vi "GetSoftwareLimits.vi"(8 "error in (no error)":errorcluster, 11 "VISA resource name":refnum<visa-resource-name>="COM15") -> (0 "error out":errorcluster, 2 "Right limit":dbl, 3 "Left limit":dbl)   [LabVIEW 2013]
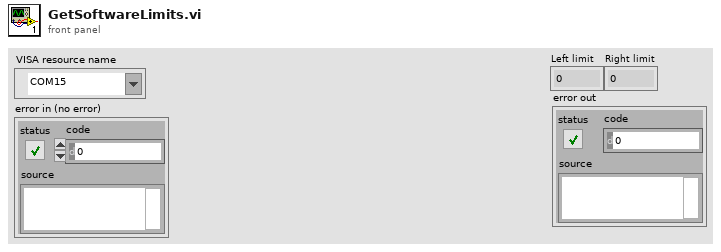
[diagram p1: front panel]
types:
  T1 = cluster{"VISA resource name":refnum<visa-resource-name>, "Device name":string, "Controller address":i32, "error":errorcluster}
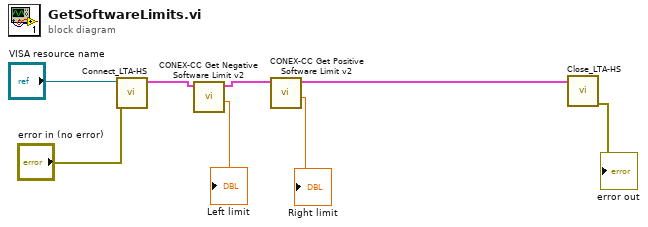
[diagram p0: block diagram]
diagram:
  n1 = call "Connect_LTA-HS.vi"("error in (no error)"="error in (no error)", "VISA resource name"="VISA resource name") -> ("Device Connection Cluster"=w7:T1)  [unwired: 8 in, 1 out]
  n2 = call "CONEX-CC Get Negative Software Limit v2.vi"("Connection Cluster in"=w7) -> ("Left limit"=→"Left limit":dbl, "Connection Cluster out"=w6:T1)  [unwired: 9 in]
  n3 = call "CONEX-CC Get Positive Software Limit v2.vi"("Connection Cluster in"=w6) -> ("Right limit"=→"Right limit":dbl, "Connection Cluster out"=w5:T1)  [unwired: 9 in]
  n4 = call "Close_LTA-HS.vi"("Connection Cluster in"=w5) -> ("error out"=→"error out":errorcluster)  [unwired: 10 in]
